vi "sv_Get Stimulus Amplitude.vi"(8 "error in (no error)":errorcluster, 10 "view":enum16{"rms", "peak", "peak-peak"}(ring), 11 "data to process":waveform(dbl)[](array[waveform])) -> (0 "error out":errorcluster, 2 "amplitude [V]":dbl, 3 "data to process out":waveform(dbl)[](array[waveform]))   [LabVIEW 2017, in "SoundVib_ContSweptSine.lvlib"]
uses:
  <vilib>/addons/Sound and Vibration/svt_Continuous Swept Sine/SoundVib_ContSweptSine.lvlib
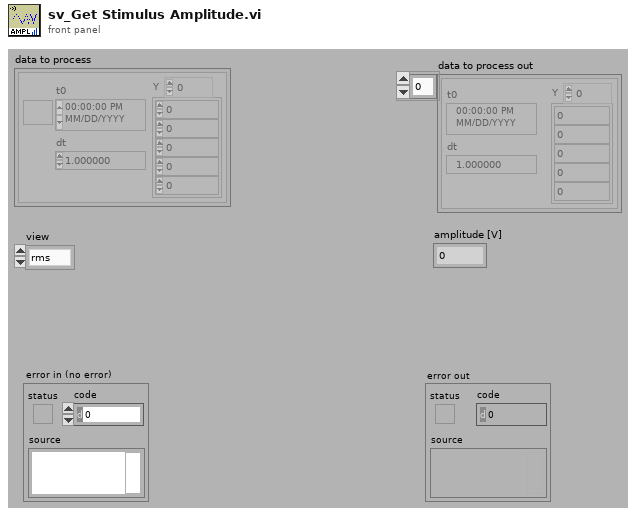
[diagram p1: front panel]
types:
  T1 = typedef "SoundVib_Generation.lvlib/sv_Chirp Settings.ctl" = cluster{"amplitude":dbl, "frequency range":cluster{"start (Hz)":dbl, "stop (Hz)":dbl, "frequency spacing":enum16{"Linear", "Logarithmic"}}, "sampling info":cluster{"Fs":dbl, "chirp duration [s]":dbl}, "initial states":cluster{"frequency [Hz]":dbl, "phase [rad]":dbl, "elapsed time [s]":dbl}, "frequency slope":dbl, "maximum harmonic":i32, "prefix len [samples]":cluster{"integer":u32, "fractional":dbl}}
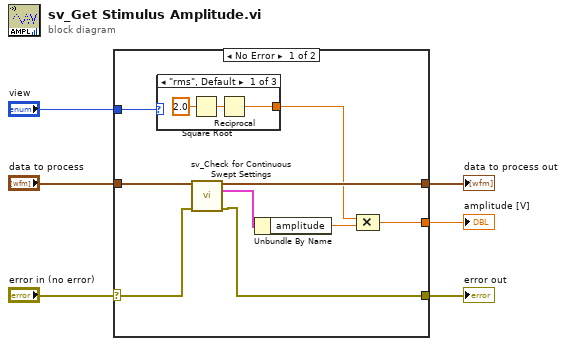
[diagram p0: block diagram]
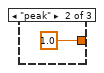
[diagram p2: hidden frame]
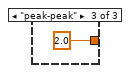
[diagram p3: hidden frame]
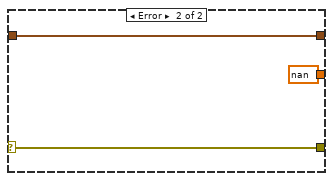
[diagram p4: hidden frame]
diagram:
  n1 = case shown="No Error" "error in (no error)" {
    selector: "error in (no error)" -> [w10 w21]
    tunnel: "data to process" -> [w13 w23]
    tunnel: [w14 w23] -> w4
    tunnel: "view" -> [w12 _]
    tunnel: [w8 nan] -> w2
    tunnel: [w7 w21] -> w1
    frame No Error {
      n2 = case shown="\"rms\", Default" w12 {
        tunnel: [w16 1.0 ("x") 2.0 ("x")] -> w9
        frame "rms", Default {
          n3 = Square Root(x=2.0) -> (sqrt(x)=w17:dbl)
          n4 = Reciprocal(x=w17) -> (1/x=w16:dbl)
        }
        frame "peak" {
        }
        frame "peak-peak" {
        }
      }
      n5 = call <vilib>:"sv_Check for Continuous Swept Settings.vi"("data to process"=w13, "error in (no error)"=w10) -> ("data to process out"=w14:waveform(dbl)[], "chirp settings"=w15:T1, "error out"=w7:errorcluster)  [unwired: 11 in]
      n6 = Unbundle By Name(w15) -> ("amplitude"=w11:dbl)
      n7 = Compound Arithmetic op=MULTIPLY(w9, w11) -> (w8:dbl)
    }
    frame Error {
    }
  }
  "error out" <- w1
  "data to process out" <- w4
  "amplitude [V]" <- w2
